vi "Get All Sequences.vi"(8 "error in (no error)":errorcluster, 11 "SequenceFile in":refnum<class "SequenceFile.lvclass">) -> (0 "error out":errorcluster, 2 "Sequences":refnum<class "Sequence.lvclass">[](array[class]), 3 "SequenceFile out":refnum<class "SequenceFile.lvclass">)   [LabVIEW 2020, in "TSnax.lvlib" / "SequenceFile.lvclass"]
uses:
  SequenceFile.lvclass
  SequenceFile.lvclass/SequenceFile.ctl
  Sequence/Sequence.lvclass
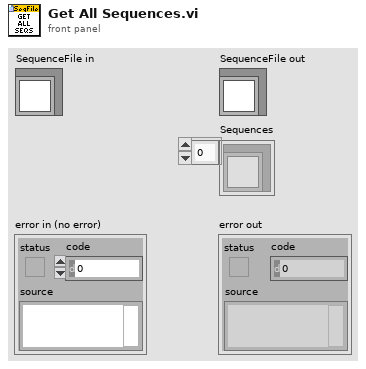
[diagram p1: front panel]
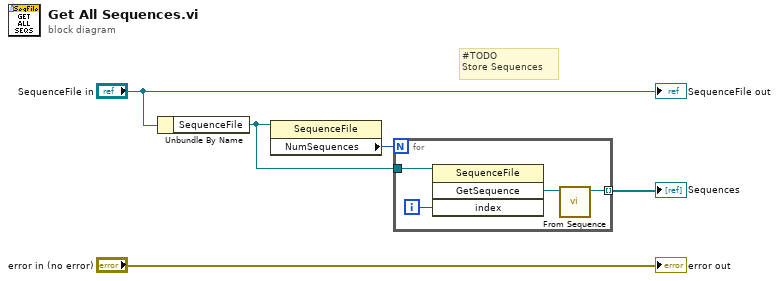
[diagram p0: block diagram]
diagram:
  # "#TODO\nStore Sequences"
  n1 = Unbundle By Name("SequenceFile in") -> ("SequenceFile"=w3:refnum<k7>)
  n2 = property class="SequenceFile"(reference=w3) -> ("NumSequences"=w2:i32)  [unwired: 1 in, 2 out]
  n3 = for {
    N: w2 -> [_]
    tunnel: w3 -> [w9]
    tunnel: [w6] -> w1 mode=indexing
    i -> [w8]
    n4 = invoke class="SequenceFile" method="GetSequence"(reference=w9, "index"=w8) -> ("GetSequence"=w7:refnum<k7>)  [unwired: 2 in, 3 out]
    n5 = call "From Sequence.vi"("Sequence"=w7) -> ("Sequence out"=w6:refnum<class "Sequence.lvclass">)  [unwired: 9 in, 1 out]
  }
  "Sequences" <- w1
  "error out" <- "error in (no error)"
  "SequenceFile out" <- "SequenceFile in"
